vi "SiosIfmInit.vi"() -> (0 "IfmInit":i32)   [LabVIEW 2009]
uses:
  siosifm.dll
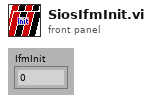
[diagram p1: front panel]
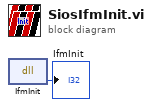
[diagram p0: block diagram]
diagram:
  n1 = dll-call lib="D:/Support/Labview/RE-10/SIOS_IfmDLL/siosifm.dll" fn="IfmInit"() -> (→"IfmInit":i32)  [unwired: 3 in, 2 out]
